vi "DebugLogger.vi"() -> ()   [LabVIEW 2010]
panel:
  out "Data":string
  in  "Clear":bool
  in  "Stop":bool
  in  "Save":bool
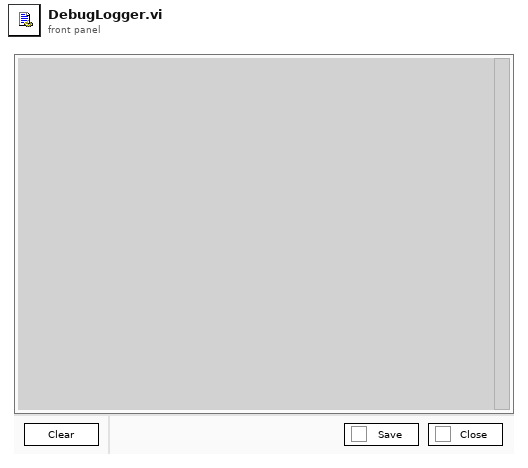
[diagram p1: front panel]
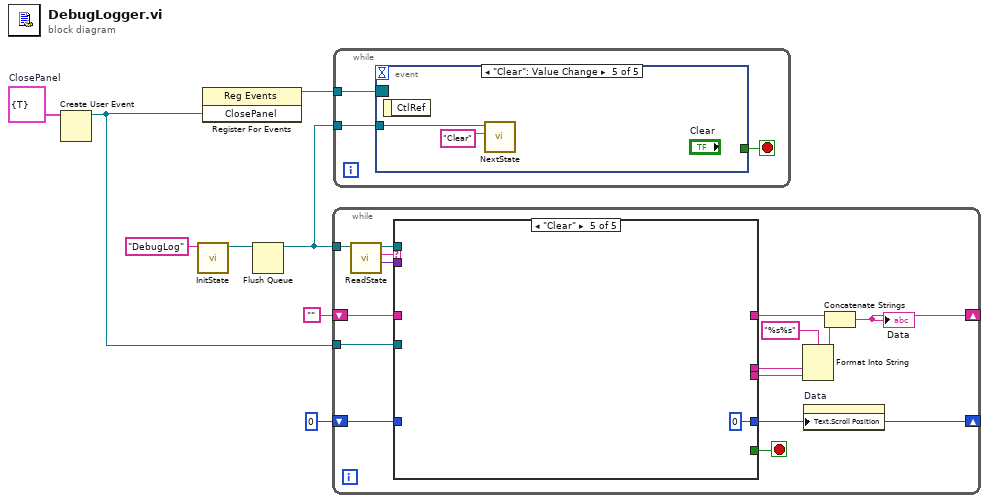
[diagram p0: block diagram]
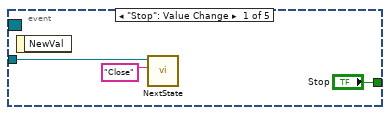
[diagram p2: hidden frame]
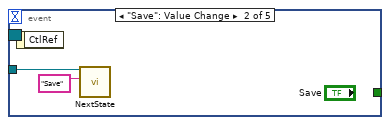
[diagram p3: hidden frame]
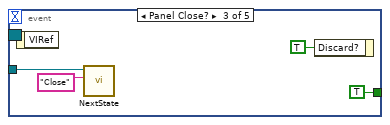
[diagram p4: hidden frame]
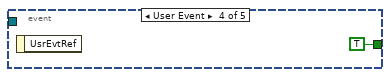
[diagram p5: hidden frame]
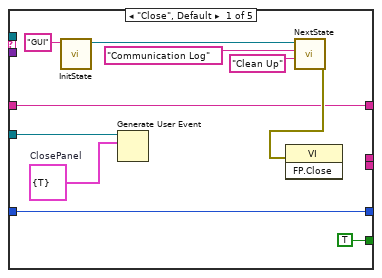
[diagram p6: hidden frame]
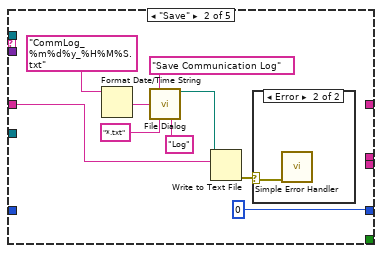
[diagram p7: hidden frame]
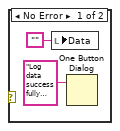
[diagram p8: hidden frame]
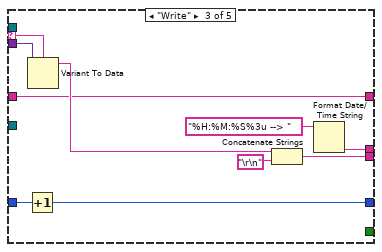
[diagram p9: hidden frame]
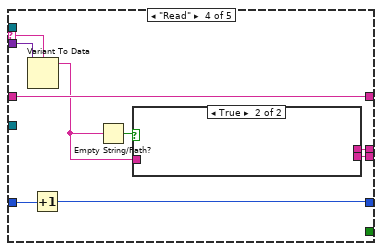
[diagram p10: hidden frame]
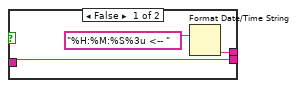
[diagram p11: hidden frame]
diagram:
  w4 = cluster{"Close":bool} {"Close"=TRUE}  # ClosePanel
  n1 = Create User Event(user event datatype=w4) -> (user event=w3:refnum<user-event>)  [unwired: 1 in, 1 out]
  n2 = call "InitState.vi"("Name"="DebugLog") -> ("Queue Out"=w7:refnum<queue>)  [unwired: 8 in, 1 out]
  n3 = register-events(w3) -> (reference out=w5:refnum<event-registration>)  [unwired: 2 in, 1 out]
  n4 = Flush Queue(queue=w7) -> (queue out=w6:refnum<queue>)  [unwired: 1 in, 2 out]
  n5 = while {
    tunnel: w6 -> [w23]
    tunnel: w3 -> [w14]
    shift-right: [w12] -> _
    shift-left: 0 -> [w13]
    shift-right: [w9] -> _
    shift-left: "" -> [w11]
    stop <- w19 stop-if-true
    n6 = call "ReadState.vi"("Queue In"=w23) -> ("Data"=w20:variant, "State"=w22:string, "Queue Out"=w21:refnum<queue>)  [unwired: 7 in, 1 out]
    n7 = case shown="\"Clear\"" w22 {
      selector: w22 -> [_ _ w54 w63 _]
      tunnel: [TRUE _ _ _ _] -> w19
      tunnel: w21 -> [_ _ _ _ _]
      tunnel: w20 -> [_ _ w55 w64 _]
      tunnel: [_ _ w52 w62 _] -> w15
      tunnel: [_ _ w49 w57 _] -> w16
      tunnel: w14 -> [w27 _ _ _ _]
      tunnel: w13 -> [w25 _ w48 w61 _]
      tunnel: [w25 0 w47 w60 0] -> w12
      tunnel: w11 -> [w24 w34 w46 w59 _]
      tunnel: [w24 _ w46 w59 _] -> w10
      frame "Close", Default {
        w26 = cluster{"Close":bool} {"Close"=TRUE}  # ClosePanel
        n8 = call "InitState.vi"("Name"="GUI") -> ("Queue Out"=w33:refnum<queue>)  [unwired: 8 in, 1 out]
        n9 = Generate User Event(user event=w27, event data cluster=w26) -> ()  [unwired: 1 in, 2 out]
        n10 = call "NextState.vi"("Data"="Clean Up" ("State"), "State"="Communication Log", "Queue In"=w33) -> ("Error Out"=w28:errorcluster)  [unwired: 7 in, 1 out]
        n11 = invoke class="VI" method="FP.Close"(error in=w28) -> ()  [unwired: 2 in, 3 out]
      }
      frame "Save" {
        n12 = Format Date/Time String(time format string (%c)="CommLog_%m%d%y_%H%M%S.txt") -> (date/time string=w36:string)  [unwired: 2 in]
        n13 = call "File Dialog"("prompt"="Save Communication Log", "default name"=w36, "pattern (all files)"="*.txt", "pattern label"="Log") -> ("selected path"=w41:path)  [unwired: 8 in, 3 out]
        n14 = Write to Text File(file (use dialog)=w41, text=w34) -> (error out=w42:errorcluster)  [unwired: 2 in, 2 out]
        n15 = case shown="Error" w42 {
          selector: w42 -> [_ w45]
          frame No Error {
            n16 = local write "Data"("") -> ()
            n17 = One Button Dialog(message="Log data successfully stored.") -> ()  [unwired: 1 in, 1 out]
          }
          frame Error {
            n18 = call <vilib>:"Simple Error Handler.vi"("error in (no error)"=w45) -> ()  [unwired: 4 in, 5 out]
          }
        }
      }
      frame "Write" {
        n19 = Increment(x=w48) -> (x+1=w47:i32)
        n20 = Variant To Data(Variant=w55, type=w54) -> (data=w51:string)  [unwired: 1 in, 1 out]
        n21 = Concatenate Strings(w51, "\r\n") -> (w49:string)
        n22 = Format Date/Time String(time format string (%c)="%H:%M:%S%3u --> ") -> (date/time string=w52:string)  [unwired: 2 in]
      }
      frame "Read" {
        n23 = Variant To Data(Variant=w64, type=w63) -> (data=w56:string)  [unwired: 1 in, 1 out]
        n24 = Increment(x=w61) -> (x+1=w60:i32)
        n25 = Empty String/Path?(string/path=w56) -> (empty?=w58:bool)
        n26 = case shown="True" w58 {
          tunnel: [w66 _] -> w62
          tunnel: w56 -> [w65 _]
          tunnel: [w65 _] -> w57
          frame False {
            n27 = Format Date/Time String(time format string (%c)="%H:%M:%S%3u <-- ") -> (date/time string=w66:string)  [unwired: 2 in]
          }
          frame True {
          }
        }
      }
      frame "Clear" {
      }
    }
    n28 = Format Into String(format string="%s%s", w15, w16) -> (resulting string=w17:string)  [unwired: 2 in, 1 out]
    n29 = property on="Data" class="Str"("Text.Scroll Position"=w12) -> ()  [unwired: 2 in, 2 out]
    n30 = Concatenate Strings(w10, w17) -> (w9:string)
    "Data" <- w9
  }
  n31 = while {
    tunnel: w6 -> [w70]
    tunnel: w5 -> [w69]
    stop <- w71 stop-if-true
    n32 = event shown="[4] \"Clear\": Value Change" {
      selector: w69 -> [_ _ _ _ _]
      dyn-events: _ -> [_ _ _ _ _]
      timeout: _ -> [_ _ _ _ _]
      tunnel: ["Stop" _ TRUE ("Stop") TRUE ("Stop") _] -> w71
      tunnel: w70 -> [w73 w75 w77 _ w82]
      event "Stop": Value Change {
        n33 = event-data() -> ()  [unwired: 1 in, 1 out]
        n34 = call "NextState.vi"("State"="Close", "Queue In"=w73) -> ()  [unwired: 8 in, 2 out]
      }
      event "Save": Value Change {
        n35 = event-data() -> ()  [unwired: 1 in, 1 out]
        n36 = call "NextState.vi"("State"="Save", "Queue In"=w75) -> ()  [unwired: 8 in, 2 out]
      }
      event Panel Close? {
        n37 = event-data() -> ()  [unwired: 1 in, 1 out]
        n38 = call "NextState.vi"("State"="Close", "Queue In"=w77) -> ()  [unwired: 8 in, 2 out]
        n39 = event-data("Discard?"=TRUE) -> ()  [unwired: 1 in, 1 out]
      }
      event User Event {
        n40 = event-data() -> ()  [unwired: 1 in, 1 out]
      }
      event "Clear": Value Change {
        n41 = event-data() -> ()  [unwired: 1 in, 1 out]
        n42 = call "NextState.vi"("State"="Clear", "Queue In"=w82) -> ()  [unwired: 8 in, 2 out]
      }
    }
  }
